vi "Configure Session.vi"(8 "error in":errorcluster, 11 "Plugin in":refnum<class "MP710995.lvclass">) -> (0 "error out":errorcluster, 3 "Plugin out":refnum<class "MP710995.lvclass">)   [LabVIEW 2025, in "MP710995.lvlib" / "MP710995.lvclass"]
uses:
  MP710995.lvclass
  C:/Program Files/National Instruments/LabVIEW 2025/vi.lib/FlexLogger/SDK/PluginSDK.lvlibp/PEFClasses/SDK/Plugin/Plugin.lvclass
  MP710995.lvclass/MP710995.ctl
  <vilib>/FlexLogger/SDK/PluginSDK.lvlibp/PEFClasses/SDK/Plugin/ParameterAccess/Write String.vi
  <vilib>/FlexLogger/SDK/PluginSDK.lvlibp/PEFClasses/SDK/Plugin/Plugin.lvclass
  <vilib>/FlexLogger/SDK/PluginSDK.lvlibp/PEFClasses/SDK/Channel/Channel.lvclass
  <vilib>/FlexLogger/SDK/PluginSDK.lvlibp/PEFClasses/SDK/Channel/ParameterAccess/Read Boolean.vi
  <vilib>/FlexLogger/SDK/PluginSDK.lvlibp/PEFClasses/SDK/Channel/ParameterAccess/Read DBL.vi
  C:/Program Files/National Instruments/LabVIEW 2025/vi.lib/FlexLogger/SDK/PluginSDK.lvlibp/PEFClasses/SDK/Processing Element/Processing Element.lvclass
  C:/Users/Steve/Documents/Git/MP710995-Plugin/Source/MP710995/MP710995.lvclass
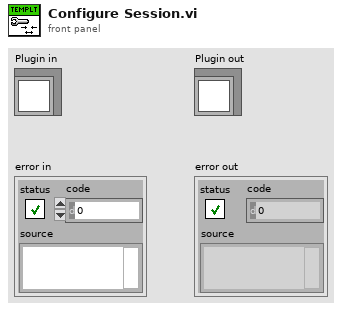
[diagram p1: front panel]
types:
  T1 = cluster{"Value":bool, "Value":dbl, "Value":dbl, "Value":bool, "Value":bool}
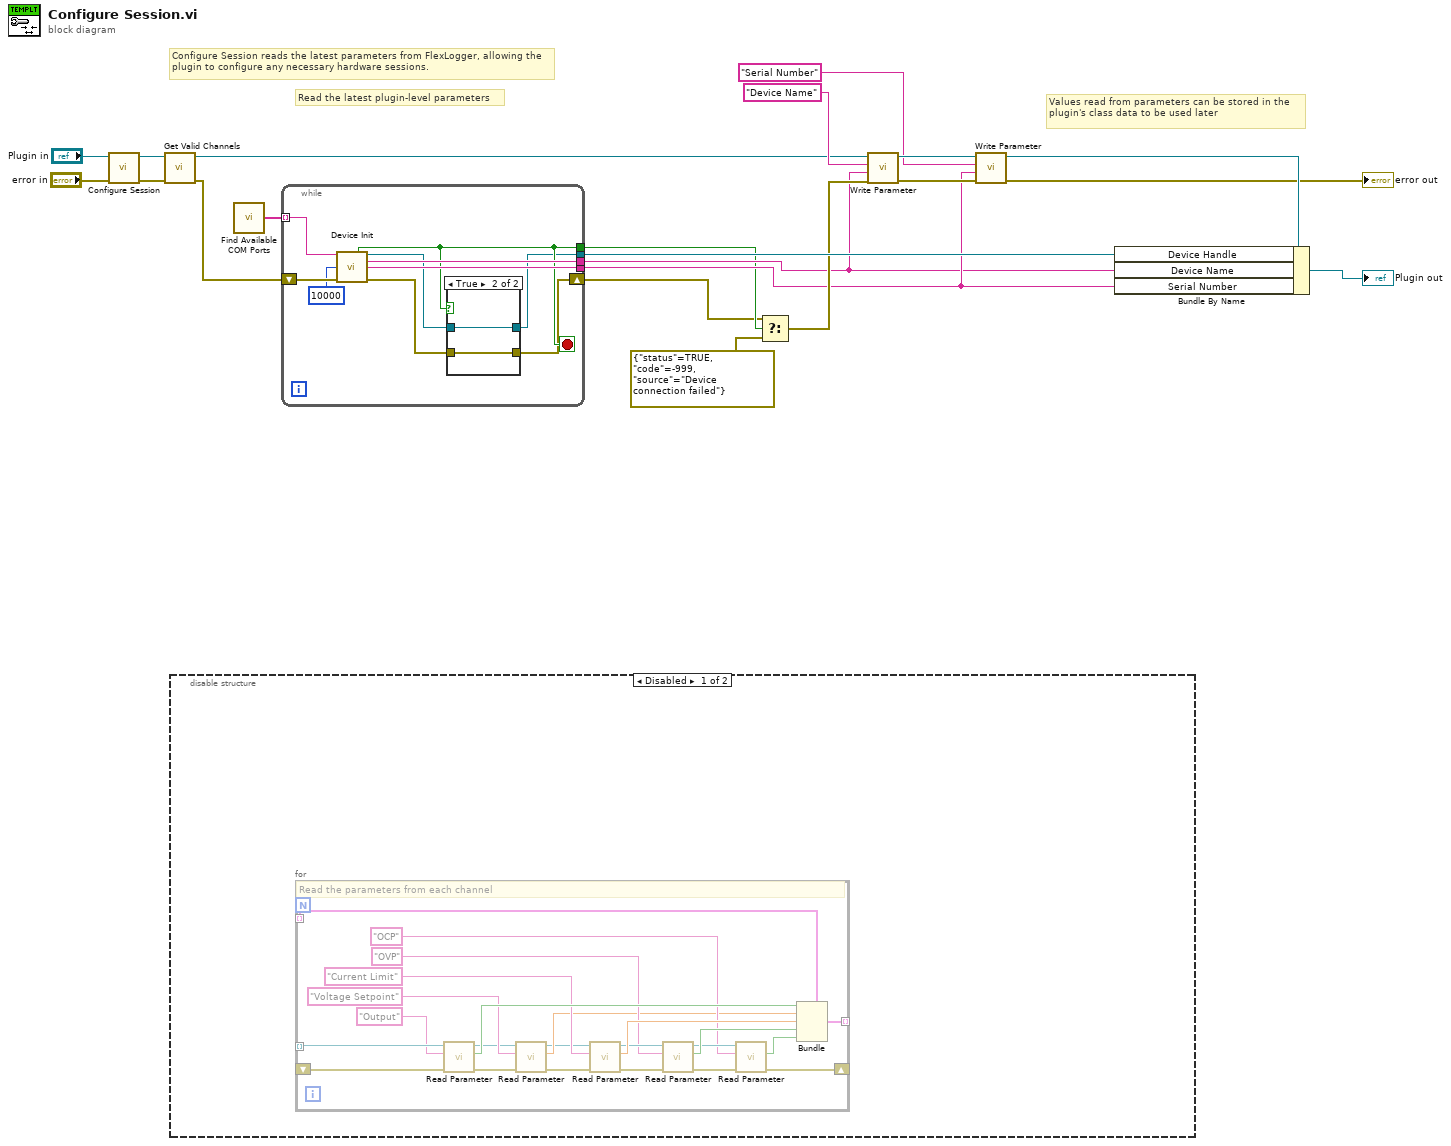
[diagram p0: block diagram]
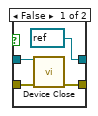
[diagram p3: hidden frame]
diagram:
  # "Read the latest plugin-level parameters"
  # "Configure Session reads the latest parameters from FlexLogger, allowing the plugin to configure any necessary hardware sessions."
  # "Values read from parameters can be stored in the plugin's class data to be used later"
  n1 = call-parent "Configure Session.vi"("error in (no error)"="error in", "Processing Element in"="Plugin in") -> ("error out"=w18:errorcluster, "Processing Element out"=w17:refnum<class "MP710995.lvclass">)  [unwired: 8 in]
  n2 = call <vilib>:"Get Valid Channels.vi"("error in (no error)"=w18, "Plugin in"=w17) -> ("error out"=w5:errorcluster, "Plugin out"=w6:refnum<class "MP710995.lvclass">)  [unwired: 7 in, 1 out]
  n3 = disable-structure shown="Disabled" {
    frame Disabled {
      n4 = for {
        tunnel: _ -> [w44] mode=indexing
        shift-right: [w40] -> _
        shift-left: _ -> [w43]
        tunnel: _ -> [w39] mode=indexing
        tunnel: [w28] -> _ mode=indexing
        # "Read the parameters from each channel"
        n5 = call-poly <vilib>:"Read Parameter.vi"("error in (no error)"=w43, "Name"="Output", "Channel in"=w44) -> ("error out"=w24:errorcluster, "Value"=w35:bool, "Channel out"=w25:refnum<class "Channel.lvclass">)  [unwired: 5 in, 1 out]
        n6 = call-poly <vilib>:"Read Parameter.vi"("error in (no error)"=w24, "Name"="Voltage Setpoint", "Channel in"=w25) -> ("error out"=w22:errorcluster, "Value"=w27:dbl, "Channel out"=w23:refnum<class "Channel.lvclass">)  [unwired: 5 in, 1 out]
        n7 = call-poly <vilib>:"Read Parameter.vi"("error in (no error)"=w22, "Name"="Current Limit", "Channel in"=w23) -> ("error out"=w42:errorcluster, "Value"=w36:dbl, "Channel out"=w34:refnum<class "Channel.lvclass">)  [unwired: 5 in, 1 out]
        n8 = call-poly <vilib>:"Read Parameter.vi"("error in (no error)"=w42, "Name"="OVP", "Channel in"=w34) -> ("error out"=w41:errorcluster, "Value"=w37:bool, "Channel out"=w33:refnum<class "Channel.lvclass">)  [unwired: 5 in, 1 out]
        n9 = call-poly <vilib>:"Read Parameter.vi"("error in (no error)"=w41, "Name"="OCP", "Channel in"=w33) -> ("error out"=w40:errorcluster, "Value"=w38:bool)  [unwired: 5 in, 2 out]
        n10 = Bundle(cluster=w39, "Value"=w35, "Value"=w27, "Value"=w36, "Value"=w37, "Value"=w38) -> (w28:T1)
      }
    }
    frame Enabled {
    }
  }
  n11 = call "Find Available COM Ports.vi"() -> ("Array"=w1:string[])  [unwired: 11 in]
  n12 = while {
    tunnel: [w45] -> w16
    tunnel: [w53] -> w8
    tunnel: [w52] -> w7
    tunnel: [w49] -> w4
    tunnel: w1 -> [w50] mode=indexing
    shift-right: [w47] -> w3
    shift-left: w5 -> [w54]
    stop <- w49 stop-if-true
    n13 = call "Device Init.vi"("Device Port"=w50, "Timeout"=u32 10000, "Error In"=w54) -> ("Connected?"=w49:bool, "VISA resource name"=w46:refnum<visa-resource-name>, "Device"=w52:string, "Serial Number"=w53:string, "Error Out"=w48:errorcluster)  [unwired: 8 in]
    n14 = case shown="True" w49 {
      tunnel: w48 -> [w58 w60]
      tunnel: [w57 w60] -> w47
      tunnel: w46 -> [w56 w59]
      tunnel: [refnum<visa-resource-name> refnum ("VISA resource name") w59] -> w45
      frame False {
        n15 = call "Device Close.vi"("VISA Rresource Name"=w56, "Error In"=w58) -> ("Error Out"=w57:errorcluster)  [unwired: 13 in]
      }
      frame True {
      }
    }
  }
  n16 = Select(t=w3, s=w4, f=errorcluster {"status"=TRUE, "code"=-999, "source"="Device connection failed"}) -> (s? t:f=w15:errorcluster)
  n17 = call-poly <vilib>:"Write Parameter.vi"("error in (no error)"=w15, "Value"=w7, "Name"="Device Name", "Plugin in"=w6) -> ("error out"=w14:errorcluster, "Plugin out"=w13:refnum<class "MP710995.lvclass">)  [unwired: 6 in]
  n18 = call-poly <vilib>:"Write Parameter.vi"("error in (no error)"=w14, "Value"=w8, "Name"="Serial Number", "Plugin in"=w13) -> ("error out"=→"error out":errorcluster, "Plugin out"=w12:refnum<class "MP710995.lvclass">)  [unwired: 6 in]
  n19 = Bundle By Name(cluster=w12, "Device Handle"=w16, "Device Name"=w7, "Serial Number"=w8) -> (→"Plugin out":refnum<class "MP710995.lvclass">)
